vi "Action list Write.vi"(4 "error in (no error)":errorcluster, 5 "Value":T2[](array[typedef]), 6 "Container State":T9, 7 "Display State In":T1) -> (0 "error out":errorcluster, 3 "Display State Out":T1)   [LabVIEW 2011, in "Action select.xctl"]
uses:
  Action select.xctl
  <vilib>/_xctls/Container State.ctl
  Action colleciton cluster.ctl
  Action common elements.ctl
  Action adjuster type.ctl
  Action type.ctl
  General command list.ctl
  PCP interface/High Level/PCP High Level Commands.ctl
  Tool/Stroker/def/Tool specific commands.ctl
  State 4.ctl
  <vilib>/_xctls/XControlSupport.lvlib
panel:
  # "Replace the Value Control below with a Control of desired type.\nDo not remove this Control or the others from the connector pane.\nDo not change the connector pane pattern.\nThe Value control should always be the third terminal from top on the input side in the connector pane."
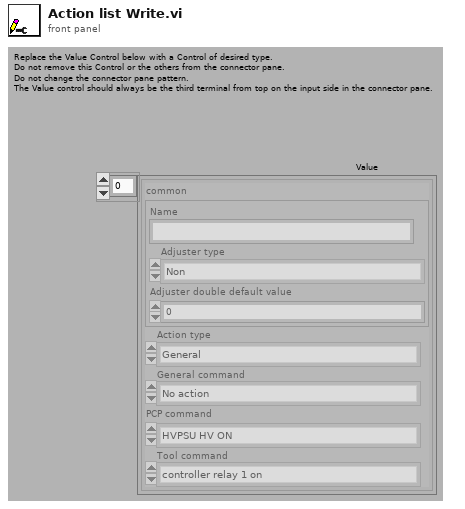
[diagram p1: front panel]
types:
  T1 = typedef "Action select.xctl/State 4.ctl" = cluster{"Actions":T2[]}
  T2 = typedef "Action colleciton cluster.ctl" = cluster{"common":T3, "Action type":T5, "General command":T6, "PCP command":T7, "Tool command":T8}
  T3 = typedef "Action common elements.ctl" = cluster{"Name":string, "Adjuster type":T4, "Adjuster double default value":dbl}
  T4 = typedef "Action adjuster type.ctl" = enum16{"Non", "Double"}
  T5 = typedef "Action type.ctl" = enum16{"General", "PCP command", "Tool command"}
  T6 = typedef "General command list.ctl" = enum16{"No action"}
  T7 = typedef "PCP High Level Commands.ctl" = enum16{"HVPSU HV ON", "HVPSU HV OFF", "PCP PC", "PCP Local", "Update Motor Voltage", "Update Cable Resistance", "Final Motor Voltage", "Final Resistance"}
  T8 = typedef "Tool specific commands.ctl" = enum16{"controller relay 1 on", "controller relay 1 off", "controller relay 2 on", "controller relay 2 off", "Solonoid 1 (master) on", "Solonoid 1 (master) off", "Solonoid 2 (Stroker) on", "Solonoid 2 (Stroker) off", "Solonoid 3 (Anchor) on", "Solonoid 3 (Anchor) off", "Controller relay 1 & 2 on", "Controller relay 1 & 2 off", "Controller relay 1 on, 2 off", "Controller relay 1 off, 2 on", "STROKER tool: Stop Force Mon", "High-G Stop", "High-G Get data", "High-G Stop Get data", "STROKER tool: Stroke out", "STROKER tool: Stroke in", "STROKER tool: Stroke stop", "STROKER tool: Stroke go to", "STROKER tool: Stop Homing", "STROKER tool: Start Force Mon dir in", "STROKER tool: Start Force Mon dir out", "Controller STOP"}
  T9 = typedef "XControlSupport.lvlib/Container State.ctl" = cluster{"Indicator?":bool, "Run Mode?":bool, " Refnum":refnum<vi>}
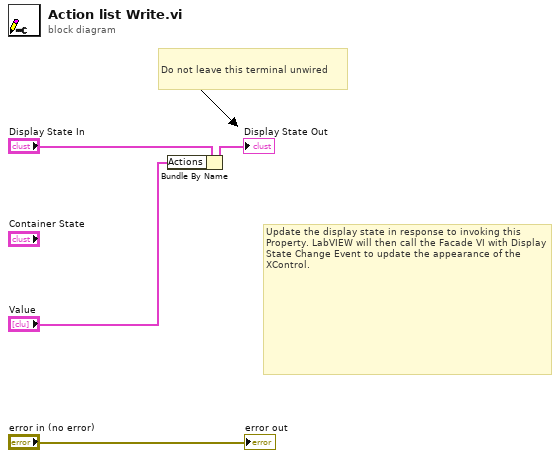
[diagram p0: block diagram]
diagram:
  # "Do not leave this terminal unwired"
  # "Update the display state in response to invoking this Property. LabVIEW will then call the Facade VI with Display State Change Event to update the appearance of the XControl."
  n1 = Bundle By Name(cluster="Display State In", "Actions"="Value") -> (→"Display State Out":T1)
  "error out" <- "error in (no error)"
